vi "write log.vi"(8 "error in (no error)":errorcluster, 10 "Event data":string, 11 "Event":string) -> (0 "error out":errorcluster)   [LabVIEW 2015]
uses:
  <vilib>/Utility/file.llb/Write Delimited Spreadsheet (string).vi
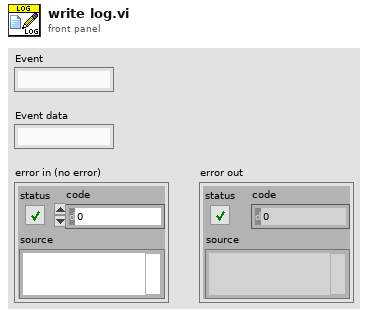
[diagram p1: front panel]
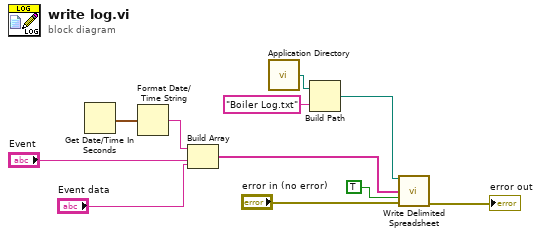
[diagram p0: block diagram]
diagram:
  n1 = Get Date/Time In Seconds() -> (seconds since 1Jan1904=w5:timestamp)
  n2 = Format Date/Time String(seconds (now)=w5) -> (date/time string=w6:string)  [unwired: 2 in]
  n3 = Build Array(w6, "Event", "Event data") -> (w9:string[])
  n4 = call <vilib>:"Application Directory.vi"() -> ("Application Directory"=w1:path)
  n5 = Build Path(base path=w1, name or relative path="Boiler Log.txt") -> (appended path=w3:path)
  n6 = call-poly <vilib>:"Write Delimited Spreadsheet.vi"("file path (dialog if empty)"=w3, "1D data"=w9, "append to file? (F)"=TRUE, "error in (no error)"="error in (no error)") -> ("error out"=→"error out":errorcluster)  [unwired: 10 in, 1 out]
